vi "Write Mapping.vi"(8 "error in (no error)":errorcluster, 10 "Mapping":T1, 11 "MLTFNC in":refnum<class "MLTFNC.lvclass">) -> (0 "error out":errorcluster, 3 "MLTFNC out":refnum<class "MLTFNC.lvclass">)   [LabVIEW 2019, in "MLTFNC.lvlib" / "MLTFNC.lvclass"]
uses:
  Library/MLTFNC.lvclass
  Custom Controls/Mapping.ctl
  Library/MLTFNC.lvclass/MLTFNC.ctl
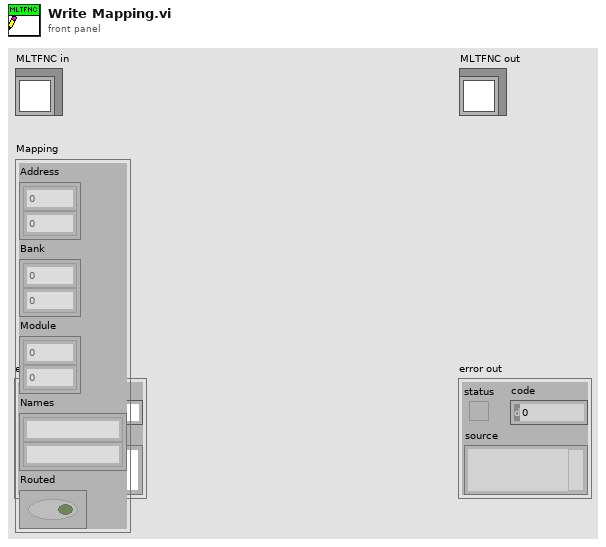
[diagram p1: front panel]
types:
  T1 = typedef "MLTFNC.lvlib/MLTFNC.lvclass/Mapping.ctl" = cluster{"Address":u32[], "Bank":u32[], "Module":u32[], "Names":string[], "Routed":bool[]}
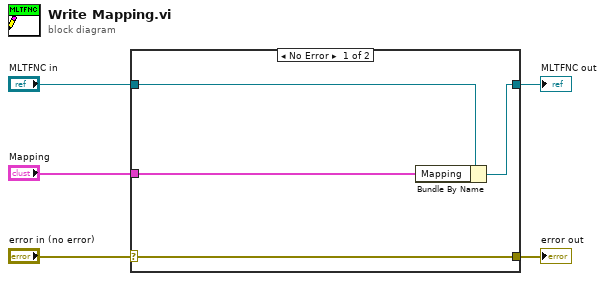
[diagram p0: block diagram]
diagram:
  n1 = case shown="No Error" "error in (no error)" {
    selector: "error in (no error)" -> [w9 w10]
    tunnel: [w9 w10] -> w4
    tunnel: [w7 w11] -> w2
    tunnel: "MLTFNC in" -> [w8 w11]
    tunnel: "Mapping" -> [w6 _]
    frame No Error {
      n2 = Bundle By Name(cluster=w8, "Mapping"=w6) -> (w7:refnum<class "MLTFNC.lvclass">)
    }
    frame Error {
    }
  }
  "error out" <- w4
  "MLTFNC out" <- w2
